vi "Write Database.vi"(8 "error in":errorcluster, 10 "Database":T1={"Baud Rate"=125000, "Frames"=[{"Name"="Frame 1", "ID"=16}, {"Name"="Frame 2", "ID"=18}]}, 11 "Path":path=path "C:/dev/niveristand-communications-bus-template/Source/Databases/DB_2F_Test.json") -> (0 "error out":errorcluster)   [LabVIEW 2020, in "Ballard MIL-STD-1553 System Explorer.lvlib" / "Implementation.lvlib"]
doc: "This VI writes a simple json database file that includes a Baud Rate and Frames where each frame includes a Name and ID."
uses:
  Implementation.lvlib
  Types/Database.ctl
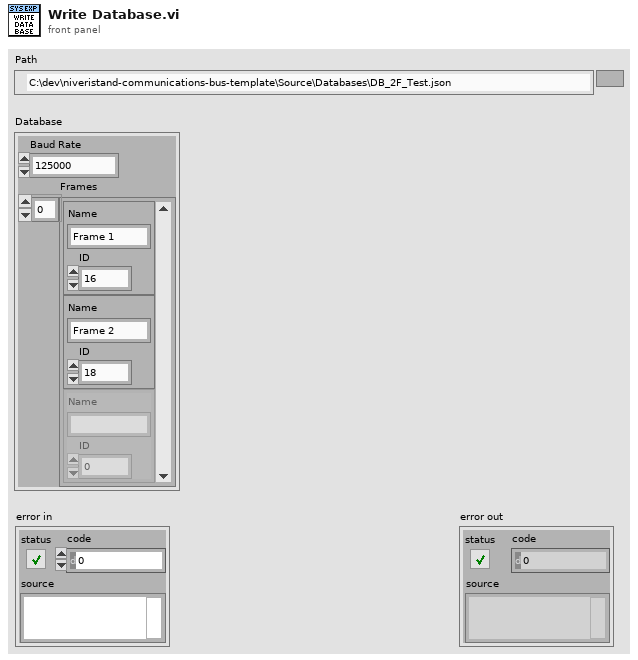
[diagram p1: front panel]
types:
  T1 = typedef "Ballard MIL-STD-1553 System Explorer.lvlib/Implementation.lvlib/Database.ctl" = cluster{"Baud Rate":u64, "Frames":cluster{"Name":string, "ID":i32}[]}
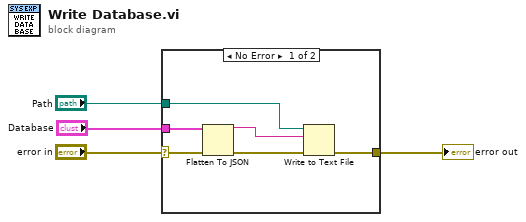
[diagram p0: block diagram]
diagram:
  n1 = case shown="No Error" "error in" {
    selector: "error in" -> [w10 w11]
    tunnel: "Database" -> [w8 _]
    tunnel: "Path" -> [w7 _]
    tunnel: [w5 w11] -> w1
    frame No Error {
      n2 = Flatten To JSON(anything=w8, error in (no error)=w10) -> (JSON string=w6:string, 11:w9:errorcluster)  [unwired: 1 in]
      n3 = Write to Text File(file (use dialog)=w7, text=w6, error in=w9) -> (error out=w5:errorcluster)  [unwired: 1 in, 2 out]
    }
    frame Error {
    }
  }
  "error out" <- w1
